vi "Init Bfr Rx - Data.vi"(7 "Data Access":refnum<class "Data Access Engine.lvclass">, 8 "error in (no error)":errorcluster, 11 "Parameters":variant) -> (0 "error out":errorcluster, 3 "Rx Loop Data":T1 {"Data Buffer" format="%016x"})   [LabVIEW 2016, in "UDP-Custom-Device Engine.lvlib"]
uses:
  UDP-Custom-Device Engine.lvlib
  <vilib>/NI/NIVS Inline Async API/_Data Access Engine/Data Access Engine/Data Access Engine.lvclass
  Types/Engine - Buffered Rx Loop Data.ctl
  Shared/Types/Shared - Header Details.ctl
  Shared/Types/Shared - Buffered.PacketInfo.ctl
  <vilib>/NI/NIVS Inline Async API/_Data Access Engine/Data Access Engine/Types/Read.DVR.ctl
  <vilib>/NI/NIVS Inline Async API/_Data Access Engine/Access Type Classes/Read/Read.lvclass
  <vilib>/NI/NIVS Inline Async API/_Data Access Engine/Data Access Engine/Types/Write.DVR.ctl
  <vilib>/NI/NIVS Inline Async API/_Data Access Engine/Access Type Classes/Write/Write.lvclass
  Shared/Types/Shared - Rx.PacketInfo.ctl
  Shared/Types/Shared - Channel Data Type.ctl
  <vilib>/NI/NIVS Inline Async API/_Data Access Engine/Data Access Engine/Methods/Write.Lookup.vi
  <vilib>/NI/NIVS Inline Async API/_Data Access Engine/Data Access Engine/Methods/Read.Lookup.vi
  Shared/UDP-Custom-Device Shared.lvlib
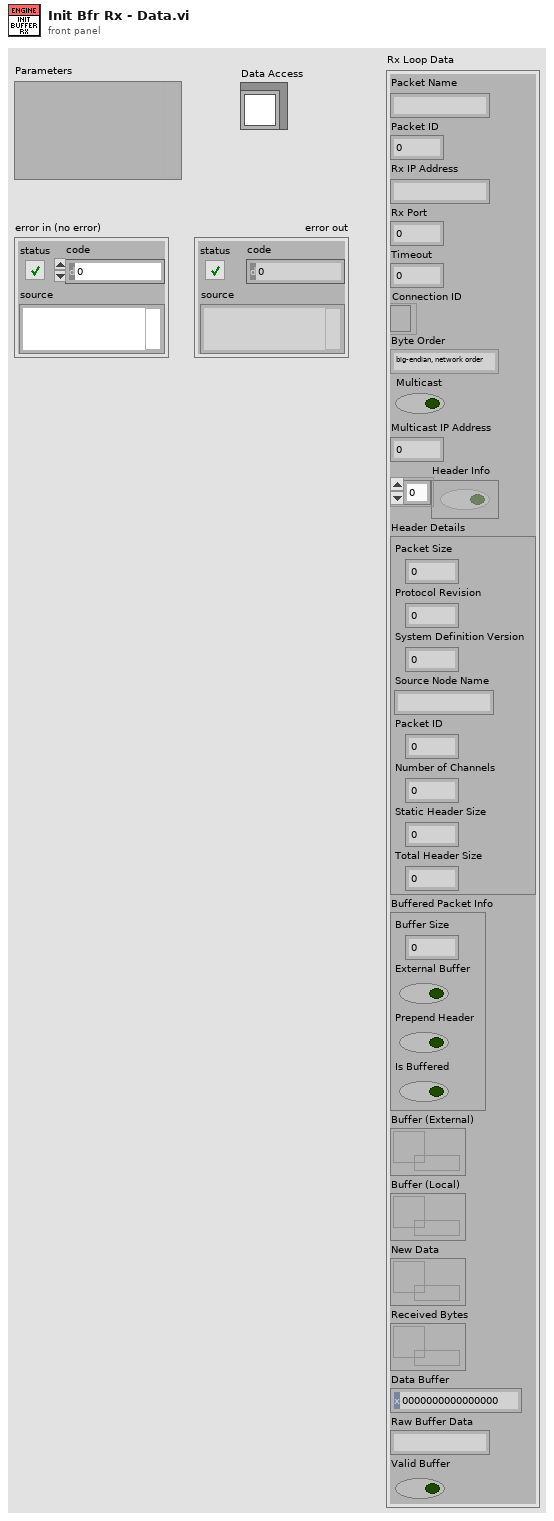
[diagram p1: front panel]
types:
  T1 = typedef "UDP-Custom-Device Engine.lvlib/Engine - Buffered Rx Loop Data.ctl" = cluster{"Packet Name":string, "Packet ID":i32, "Rx IP Address":string, "Rx Port":i32, "Timeout":i32, "Connection ID":refnum<k16>, "Byte Order":enum16{"big-endian, network order", "native, host order", "little-endian"}, "Multicast":bool, "Multicast IP Address":u32, "Header Info":bool[], "Header Details":T2, "Buffered Packet Info":T3, "Buffer (External)":T4, "Buffer (Local)":T5, "New Data":T5, "Received Bytes":T5, "Data Buffer":u64, "Raw Buffer Data":string, "Valid Buffer":bool}
  T2 = typedef "UDP-Custom-Device Shared.lvlib/Shared - Header Details.ctl" = cluster{"Packet Size":u16, "Protocol Revision":u8, "System Definition Version":u64, "Source Node Name":string, "Packet ID":u32, "Number of Channels":u32, "Static Header Size":u16, "Total Header Size":u16}
  T3 = typedef "UDP-Custom-Device Shared.lvlib/Shared - Buffered.PacketInfo.ctl" = cluster{"Buffer Size":i32, "External Buffer":bool, "Prepend Header":bool, "Is Buffered":bool}
  T4 = typedef "Data Access Engine.lvlib/Data Access Engine.lvclass/Read.DVR.ctl" = refnum<data-value>
  T5 = typedef "Data Access Engine.lvlib/Data Access Engine.lvclass/Write.DVR.ctl" = refnum<data-value>
  T6 = typedef "UDP-Custom-Device Shared.lvlib/Shared - Rx.PacketInfo.ctl" = cluster{"Packet Name":string, "Packet ID":i32, "Timeout":i32, "Rx IP Address":string, "Rx Port":u16, "Endianness":u16, "Multicast":bool, "Multicast IP Address":string, "Diagnostics En?":bool, "Header Info":bool[], "Channel Data Types":T7[], "Buffered Packet Info":T3}
  T7 = typedef "UDP-Custom-Device Shared.lvlib/Shared - Channel Data Type.ctl" = enum16{"Boolean", "Single", "Double", "I8", "I16", "I32", "I64", "U8", "U16", "U32", "U64"}
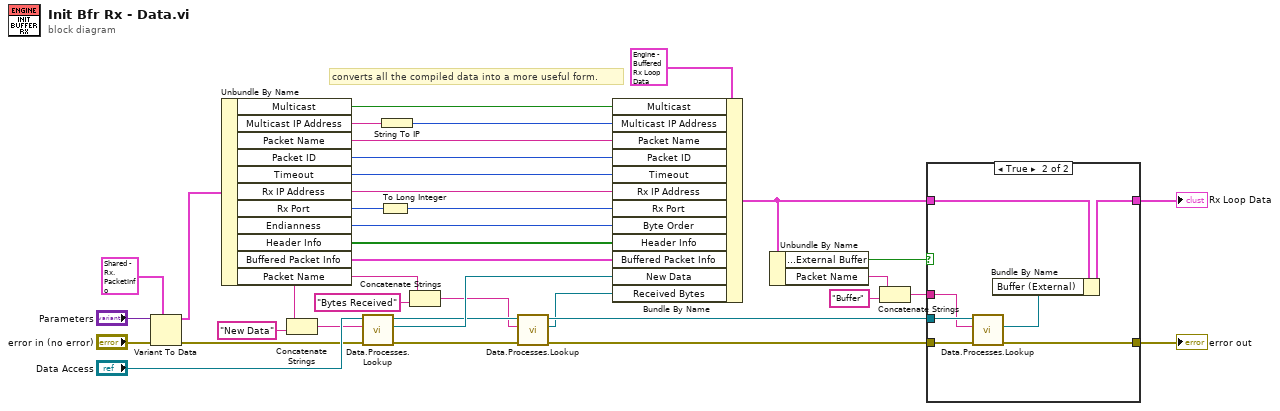
[diagram p0: block diagram]
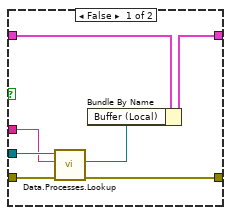
[diagram p2: hidden frame]
diagram:
  # "converts all the compiled data into a more useful form."
  n1 = Variant To Data(error in="error in (no error)", type=T6 {"Packet Name"="", "Packet ID"=0, "Timeout"=0, "Rx IP Address"="", "Rx Port"=0, "Endianness"=0, "Multicast"=FALSE, "Multicast IP Address"="", "Diagnostics En?"=FALSE, "Header Info"=[], "Channel Data Types"=[], "Buffered Packet Info"={"Buffer Size"=0, "External Buffer"=FALSE, "Prepend Header"=FALSE, "Is Buffered"=FALSE}} ("Rx Packet Info"), Variant="Parameters") -> (data=w34:T6, error out=w16:errorcluster)
  n2 = Unbundle By Name(w34) -> ("Multicast"=w11:bool, "Multicast IP Address"=w10:string, "Packet Name"=w32:string, "Packet ID"=w31:i32, "Timeout"=w12:i32, "Rx IP Address"=w30:string, "Rx Port"=w29:u16, "Endianness"=w27:u16, "Header Info"=w26:bool[], "Buffered Packet Info"=w25:T3, "Packet Name"=w4:string)
  n3 = Concatenate Strings(w4, "New Data" ("Item GUID")) -> (w14:string)
  n4 = call-poly <vilib>:"Data.Processes.Lookup.vi"("error in (no error)"=w16, "Name"=w14, "Data Access API in"="Data Access") -> ("error out"=w6:errorcluster, "Ref"=w13:T5, "Data Access API out"=w8:refnum<class "Data Access Engine.lvclass">)  [unwired: 5 in, 1 out]
  n5 = To Long Integer(number=w29) -> (32bit integer=w28:i32)
  n6 = String To IP(1:w10) -> (0:w9:u32)
  n7 = Concatenate Strings(w4, "Bytes Received" ("string")) -> (w2:string)
  n8 = call-poly <vilib>:"Data.Processes.Lookup.vi"("error in (no error)"=w6, "Name"=w2, "Data Access API in"=w8) -> ("error out"=w5:errorcluster, "Ref"=w1:T5, "Data Access API out"=w7:refnum<class "Data Access Engine.lvclass">)  [unwired: 5 in, 1 out]
  n9 = Bundle By Name(cluster=T1 {"Packet Name"="", "Packet ID"=0, "Rx IP Address"="", "Rx Port"=0, "Timeout"=0, "Connection ID"=refnum, "Byte Order"=enum."big-endian, network order", "Multicast"=FALSE, "Multicast IP Address"=0, "Header Info"=[], "Header Details"={"Packet Size"=0, "Protocol Revision"=0, "System Definition Version"=0, "Source Node Name"="", "Packet ID"=0, "Number of Channels"=0, "Static Header Size"=0, "Total Header Size"=0}, "Buffered Packet Info"={"Buffer Size"=0, "External Buffer"=FALSE, "Prepend Header"=FALSE, "Is Buffered"=FALSE}, "Buffer (External)"=refnum, "Buffer (Local)"=refnum, "New Data"=refnum, "Received Bytes"=refnum, "Data Buffer"=0, "Raw Buffer Data"="", "Valid Buffer"=FALSE} ("Rx Loop Data"), "Multicast"=w11, "Multicast IP Address"=w9, "Packet Name"=w32, "Packet ID"=w31, "Timeout"=w12, "Rx IP Address"=w30, "Rx Port"=w28, "Byte Order"=w27, "Header Info"=w26, "Buffered Packet Info"=w25, "New Data"=w13, "Received Bytes"=w1) -> (w20:T1)
  n10 = Unbundle By Name(w20) -> ("Buffered Packet Info.External Buffer"=w22:bool, "Packet Name"=w23:string)
  n11 = Concatenate Strings(w23, "Buffer" ("Item GUID")) -> (w24:string)
  n12 = case shown="True" w22 {
    tunnel: [w40 w47] -> w19
    tunnel: w20 -> [w41 w48]
    tunnel: [w38 w45] -> w18
    tunnel: w5 -> [w39 w46]
    tunnel: w7 -> [w44 w51]
    tunnel: w24 -> [w43 w50]
    frame False {
      n13 = call-poly <vilib>:"Data.Processes.Lookup.vi"("error in (no error)"=w39, "Name"=w43, "Data Access API in"=w44) -> ("error out"=w38:errorcluster, "Ref"=w42:T5)  [unwired: 5 in, 2 out]
      n14 = Bundle By Name(cluster=w41, "Buffer (Local)"=w42) -> (w40:T1)
    }
    frame True {
      n15 = call-poly <vilib>:"Data.Processes.Lookup.vi"("error in (no error)"=w46, "Name"=w50, "Data Access API in"=w51) -> ("error out"=w45:errorcluster, "Ref"=w49:T4)  [unwired: 5 in, 2 out]
      n16 = Bundle By Name(cluster=w48, "Buffer (External)"=w49) -> (w47:T1)
    }
  }
  "error out" <- w18
  "Rx Loop Data" <- w19
